vi "Initialise montage canvas.vi"(6 "Image bitness":enum16{"8bit", "16bit"}(ring), 8 "Error in":errorcluster, 10 "Number of rows to generate":i32=6, 11 "Experiment Parameters":T3) -> (0 "error out":errorcluster, 1 "Rows/Columns":T2={"Number of rows to generate"=6, "Number of columns to generate"=0}, 2 "U8 Image ref (Montage)":T1, 3 "I16 Image ref (Montage)":T1)   [LabVIEW 2020]
uses:
  <vilib>/vision/Image Controls.llb/IMAQ Image.ctl
  Typedefs/Experiment Parameters.ctl
panel:
  out "Y Resolution of collage":i32
  out "X Resolution of collage":i32
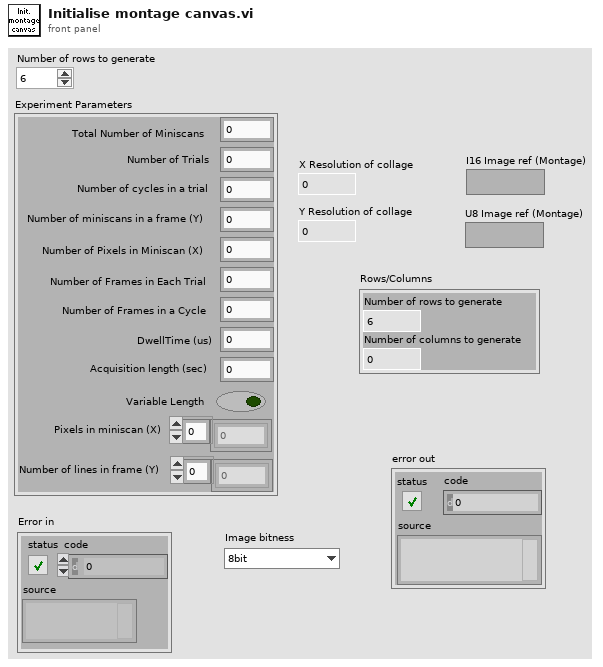
[diagram p1: front panel]
types:
  T1 = typedef "IMAQ Image.ctl" = refnum<image>
  T2 = cluster{"Number of rows to generate":i32, "Number of columns to generate":i32}
  T3 = typedef "Experiment Parameters.ctl" = cluster{"Total Number of Miniscans":i32, "Number of Trials":i32, "Number of cycles in a trial":i32, "Number of miniscans in a frame (Y)":i32, "Number of Pixels in Miniscan (X)":i32, "Number of Frames in Each Trial":i32, "Number of Frames in a Cycle":i32, "DwellTime (us)":dbl, "Acquisition length (sec)":dbl, "Variable Length":bool, "Pixels in miniscan (X)":dbl[], "Number of lines in frame (Y)":dbl[]}
  T4 = typedef "Image Type" = u32
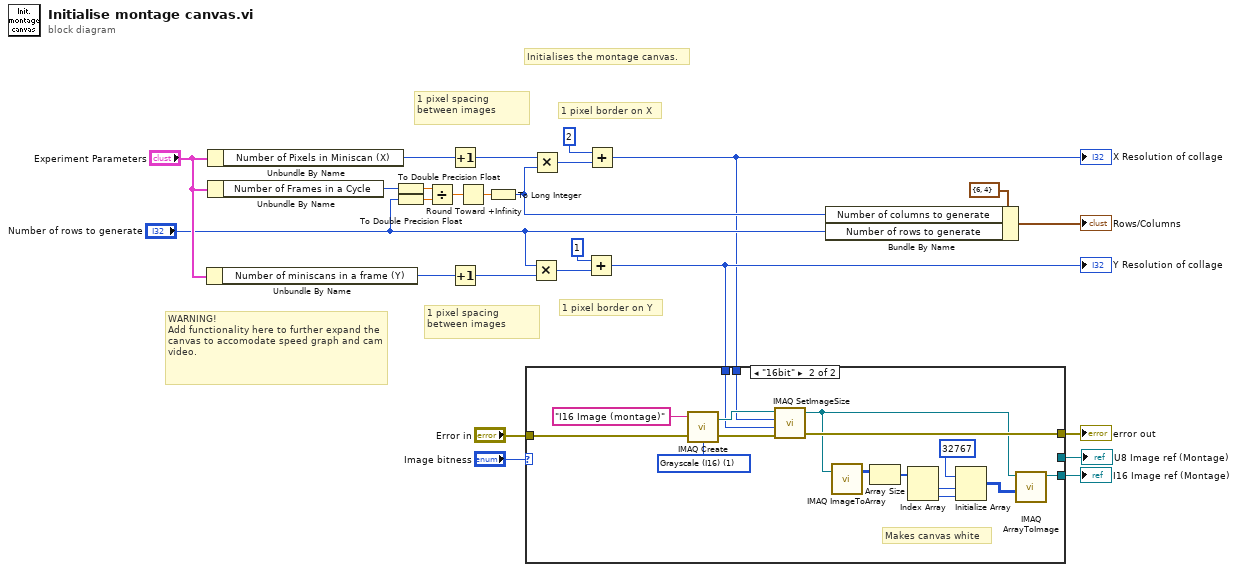
[diagram p0: block diagram]
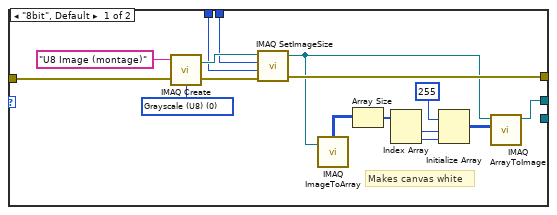
[diagram p2: hidden frame]
diagram:
  # "1 pixel border on X"
  # "1 pixel border on Y"
  # "1 pixel spacing between images"
  # "1 pixel spacing between images"
  # "WARNING!\nAdd functionality here to further expand the canvas to accomodate speed graph and cam video."
  # "Initialises the montage canvas."
  n1 = Unbundle By Name("Experiment Parameters") -> ("Number of miniscans in a frame (Y)"=w17:i32)
  n2 = Unbundle By Name("Experiment Parameters") -> ("Number of Pixels in Miniscan (X)"=w20:i32)
  n3 = Unbundle By Name("Experiment Parameters") -> ("Number of Frames in a Cycle"=w24:i32)
  n4 = To Double Precision Float(number=w24) -> (double precision float=w22:dbl)
  n5 = To Double Precision Float(number="Number of rows to generate") -> (double precision float=w21:dbl)
  n6 = Divide(x=w22, y=w21) -> (x/y=w23:dbl)
  n7 = Increment(x=w20) -> (x+1=w9:i32)
  n8 = Increment(x=w17) -> (x+1=w10:i32)
  n9 = Round Toward +Infinity(x=w23) -> (ceil(x): smallest int >= x=w25:dbl)
  n10 = To Long Integer(number=w25) -> (32bit integer=w12:i32)
  n11 = Multiply(x="Number of rows to generate", y=w10) -> (x*y=w8:i32)
  n12 = Multiply(x=w9, y=w12) -> (x*y=w19:i32)
  n13 = Add(x=1, y=w8) -> (x+y=w7:i32)
  "Y Resolution of collage" <- w7
  n14 = Add(x=2, y=w19) -> (x+y=w6:i32)
  "X Resolution of collage" <- w6
  n15 = case shown="\"16bit\"" "Image bitness" {
    tunnel: [w37 w53] -> w16
    tunnel: [_ w51] -> w11
    tunnel: w7 -> [w35 w50]
    tunnel: w6 -> [w34 w49]
    tunnel: "Error in" -> [w27 w44]
    tunnel: [w26 _] -> w1
    frame "8bit", Default {
      w40 = T4 0 items=["Grayscale (U8)", "Grayscale (I16)", "Grayscale (SGL)", "Complex (CSG)", "RGB (U32)", "HSL (U32)", "RGB (U64)", "Grayscale (U16)"] ("Image Type")
      # "Makes canvas white"
      n16 = call "IMAQ Create"("Image Name"="U8 Image (montage)", "Image Type"=w40, "error in (no error)"=w27) -> ("New Image"=w39:T1, "error out"=w38:errorcluster)  [unwired: 1 in, 1 out]
      n17 = call "IMAQ SetImageSize"("error in (no error)"=w38, "Y Resolution"=w35, "X Resolution"=w34, "Image"=w39) -> ("error out"=w37:errorcluster, "Image Out"=w36:T1)  [unwired: 1 out]
      n18 = call "IMAQ ImageToArray"("Image"=w36) -> ("Image Pixels (U8)"=w29:u8[][])  [unwired: 3 in, 4 out]
      n19 = Array Size(array=w29) -> (size(s)=w33:i32[])
      n20 = Index Array(array=w33) -> (element #1=w32:i32, element #2=w31:i32)  [unwired: 2 in]
      n21 = Initialize Array(u8 255, w32, w31) -> (w28:u8[][])
      n22 = call "IMAQ ArrayToImage"("Image Pixels (U8)"=w28, "Image"=w36) -> ("Image Out"=w26:T1)  [unwired: 8 in, 1 out]
    }
    frame "16bit" {
      w56 = T4 1 items=["Grayscale (U8)", "Grayscale (I16)", "Grayscale (SGL)", "Complex (CSG)", "RGB (U32)", "HSL (U32)", "RGB (U64)", "Grayscale (U16)"] ("Image Type")
      # "Makes canvas white"
      n23 = call "IMAQ Create"("Image Name"="I16 Image (montage)", "Image Type"=w56, "error in (no error)"=w44) -> ("New Image"=w55:T1, "error out"=w54:errorcluster)  [unwired: 1 in, 1 out]
      n24 = call "IMAQ SetImageSize"("error in (no error)"=w54, "Y Resolution"=w50, "X Resolution"=w49, "Image"=w55) -> ("error out"=w53:errorcluster, "Image Out"=w52:T1)  [unwired: 1 out]
      n25 = call "IMAQ ImageToArray"("Image"=w52) -> ("Image Pixels (I16)"=w42:i16[][])  [unwired: 3 in, 4 out]
      n26 = Array Size(array=w42) -> (size(s)=w48:i32[])
      n27 = Index Array(array=w48) -> (element #1=w47:i32, element #2=w46:i32)  [unwired: 2 in]
      n28 = Initialize Array(i16 32767, w47, w46) -> (w43:i16[][])
      n29 = call "IMAQ ArrayToImage"("Image Pixels (I16)"=w43, "Image"=w52) -> ("Image Out"=w51:T1)  [unwired: 8 in, 1 out]
    }
  }
  "I16 Image ref (Montage)" <- w11
  "error out" <- w16
  "U8 Image ref (Montage)" <- w1
  n30 = Bundle By Name(cluster=T2 {"Number of rows to generate"=6, "Number of columns to generate"=4} ("Rows/Columns"), "Number of columns to generate"=w12, "Number of rows to generate"="Number of rows to generate") -> (→"Rows/Columns":T2)
